vi "get folder size and file count.vi"(11 "Path":path) -> (1 "Number of Files":i32, 3 "size":i64)   [LabVIEW 2023]
panel:
  out "error out":errorcluster
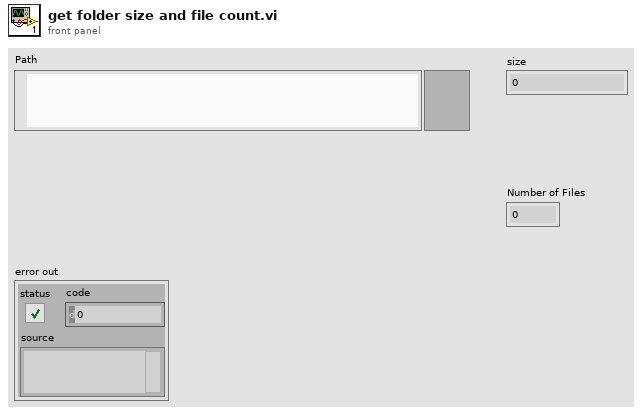
[diagram p1: front panel]
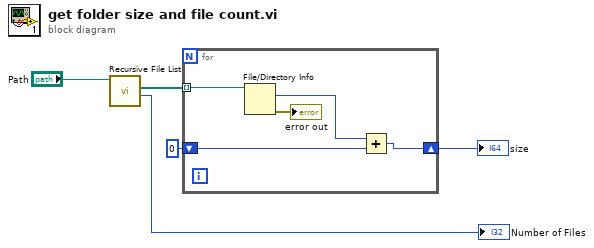
[diagram p0: block diagram]
diagram:
  n1 = call <vilib>:"Recursive File List.vi"("Folder Path"="Path") -> ("Number of Files"=→"Number of Files":i32, "All Files in Dir"=w4:path[])  [unwired: 6 in, 3 out]
  n2 = for {
    tunnel: w4 -> [w10] mode=indexing
    shift-right: [w8] -> w2
    shift-left: i64 0 ("size") -> [w7]
    n3 = File/Directory Info(path=w10) -> (size=w9:i64, error out=→"error out":errorcluster)  [unwired: 1 in, 5 out]
    n4 = Add(x=w9, y=w7) -> (x+y=w8:i64)
  }
  "size" <- w2
